vi "stop.vi"(8 "error in (no error)":errorcluster, 11 "HGF_DSCVarManager in":refnum<class "HGF_DSCVarManager.lvclass">) -> (0 "error out":errorcluster, 3 "HGF_DSCVarManager out":refnum<class "HGF_DSCVarManager.lvclass">)   [LabVIEW 2012, in "HGF_DSC.lvlib" / "HGF_DSCVarManager.lvclass"]
uses:
  HGF_DSCVarManager.lvclass
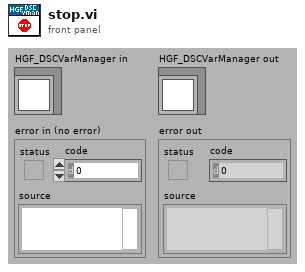
[diagram p1: front panel]
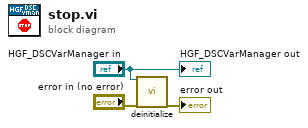
[diagram p0: block diagram]
diagram:
  n1 = call-dynamic "deinitialize.vi"("HGF_DSCVarManager"="HGF_DSCVarManager in", "error in (no error)"="error in (no error)") -> ("error out"=→"error out":errorcluster)  [unwired: 17 in]
  "HGF_DSCVarManager out" <- "HGF_DSCVarManager in"
